vi "Test_Cuboid_Math.vi"() -> ()   [LabVIEW 2023]
uses:
  3Dpoint.ctl
  3DCuboid.ctl
panel:
  out "PointIsInsideCuboid":bool
  out "Output Point":T1
  out "Nearest Point":T1
  in  "Z":dbl
  in  "Y":dbl
  in  "X":dbl
  in  "OriginZ":dbl
  in  "OriginY":dbl
  in  "OriginX":dbl
  in  "Height(Z)":dbl
  in  "Width(Y)":dbl
  in  "Length(X)":dbl
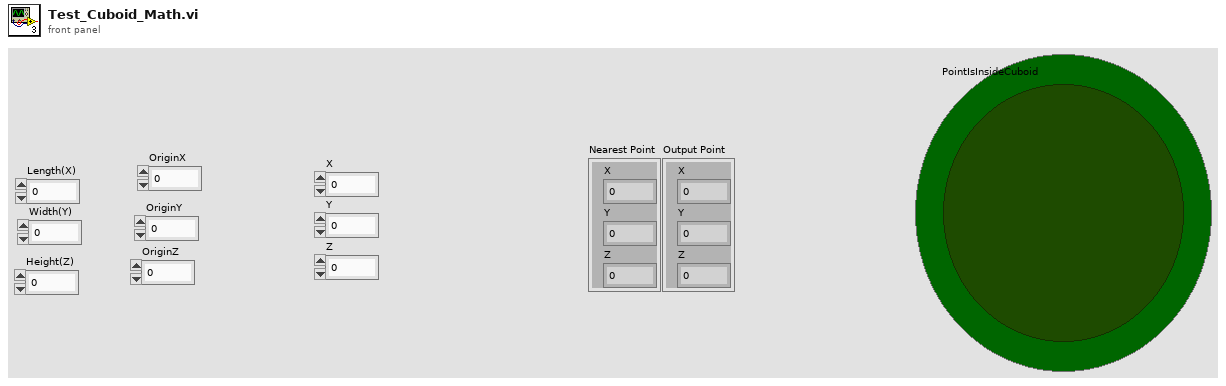
[diagram p1: front panel]
types:
  T1 = typedef "3Dpoint.ctl" = cluster{"X":dbl, "Y":dbl, "Z":dbl}
  T2 = typedef "3DCuboid.ctl" = cluster{"Length(X)":dbl, "Width(Y)":dbl, "Height(Z)":dbl, "OriginPoint":T1}
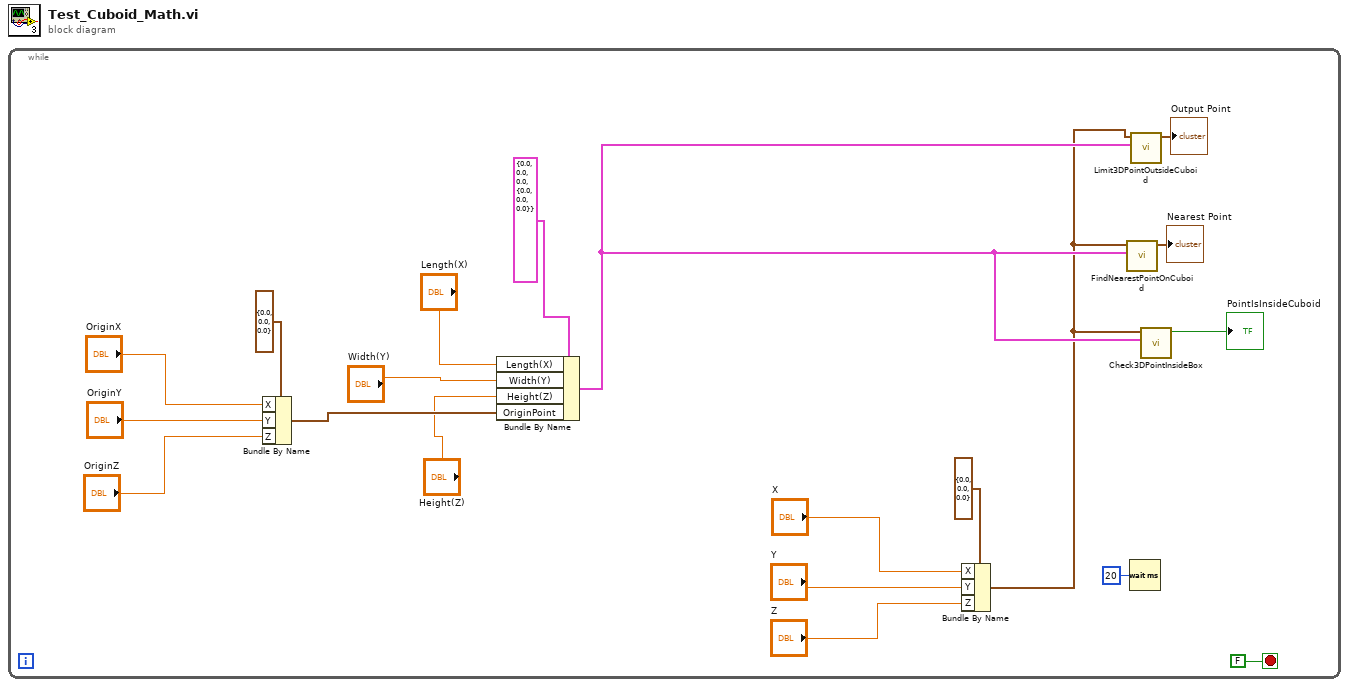
[diagram p0: block diagram]
diagram:
  n1 = while {
    stop <- FALSE stop-if-true
    n2 = Bundle By Name(cluster=T1 {"X"=0.0, "Y"=0.0, "Z"=0.0} ("3D Point"), "X"="OriginX", "Y"="OriginY", "Z"="OriginZ") -> (w18:T1)
    n3 = Bundle By Name(cluster=T2 {"Length(X)"=0.0, "Width(Y)"=0.0, "Height(Z)"=0.0, "OriginPoint"={"X"=0.0, "Y"=0.0, "Z"=0.0}} ("3D Cuboid"), "Length(X)"="Length(X)", "Width(Y)"="Width(Y)", "Height(Z)"="Height(Z)", "OriginPoint"=w18) -> (w3:T2)
    n4 = Bundle By Name(cluster=T1 {"X"=0.0, "Y"=0.0, "Z"=0.0} ("3D Point"), "X"="X", "Y"="Y", "Z"="Z") -> (w2:T1)
    n5 = call "FindNearestPointOnCuboid.vi"("3D Cuboid"=w3, "3D Point"=w2) -> ("Nearest Point"=→"Nearest Point":T1)  [unwired: 9 in]
    n6 = Wait (ms)(milliseconds to wait=u32 20) -> ()  [unwired: 1 out]
    n7 = call "Limit3DPointOutsideCuboid.vi"("3D Cuboid"=w3, "3D Point"=w2) -> ("Output Point"=→"Output Point":T1)  [unwired: 9 in]
    n8 = call "Check3DPointInsideBox.vi"("3D Cuboid"=w3, "3D Point"=w2) -> ("PointIsInsideCuboid"=→"PointIsInsideCuboid":bool)  [unwired: 9 in]
  }
